vi "Save_Spectrum.vi"(2 "button on":bool, 3 "averaging complete":bool) -> (0 "button on":bool, 1 "save spectrum":bool)   [LabVIEW 2013]
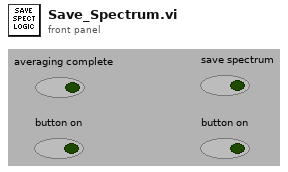
[diagram p1: front panel]
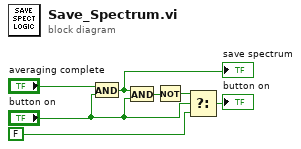
[diagram p0: block diagram]
diagram:
  n1 = And(x="averaging complete", y="button on") -> (x .and. y?=w2:bool)
  "save spectrum" <- w2
  n2 = And(x=w2, y="button on") -> (x .and. y?=w7:bool)
  n3 = Not(x=w7) -> (.not. x?=w6:bool)
  n4 = Select(t=w6, s="button on", f=FALSE) -> (s? t:f=→"button on":bool)
